vi "Auto Launch.vi"(8 "error in (no error)":errorcluster, 11 "Task in":refnum<class "Task Config.lvclass">) -> (0 "error out":errorcluster, 2 "Auto Launch":bool, 3 "Task out":refnum<class "Task Config.lvclass">)   [LabVIEW 2020, in "VolatusConfig.lvlib" / "Task Config.lvclass"]
uses:
  Task Config.lvclass
  Task Config.lvclass/Task Config.ctl
  lv-cdm/CDM-Config/Config Element/Config Element.lvclass
  VolatusConfigElement/VolatusConfigElement.lvclass
  C:/dev/lv20CE/relink/lv-volatus/VolatusConfig/VolatusConfigElement/VolatusConfigElement.lvclass
  C:/dev/lv20CE/relink/lv-volatus/VolatusConfig/Task/Task Config.lvclass
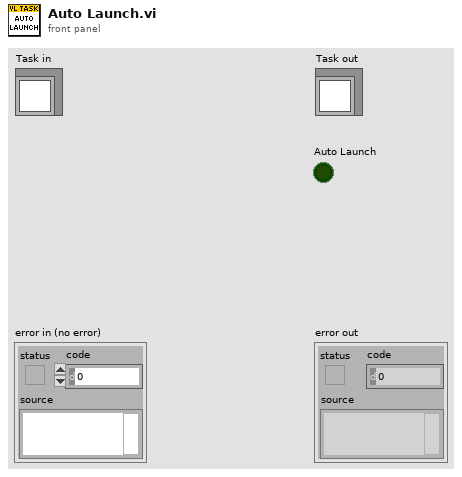
[diagram p1: front panel]
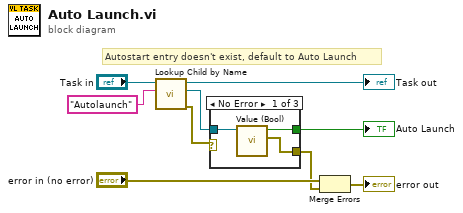
[diagram p0: block diagram]
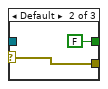
[diagram p2: hidden frame]
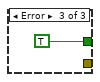
[diagram p3: hidden frame]
diagram:
  # "Autostart entry doesn't exist, default to Auto Launch"
  n1 = call "Lookup Child by Name.vi"("Child Name"="Autolaunch" ("Name"), "VolatusConfigElement in"="Task in") -> ("error out"=w2:errorcluster, "Child"=w1:refnum<class "Config Element.lvclass">, "VolatusConfigElement out"=→"Task out":refnum<class "Task Config.lvclass">)  [unwired: 6 in, 1 out]
  n2 = case shown="No Error" w2 {
    selector: w2 -> [_ w13 _]
    tunnel: [w11 FALSE ("Bool Value") TRUE] -> w7
    tunnel: w1 -> [w12 _ _]
    tunnel: [w10 w13 _] -> w5
    frame No Error {
      n3 = call "Value (Bool).vi"("Config Element in"=w12) -> ("error out"=w10:errorcluster, "Bool Value"=w11:bool)  [unwired: 9 in]
    }
    frame Default {
    }
    frame Error {
    }
  }
  "Auto Launch" <- w7
  n4 = Merge Errors("error in (no error)", w5) -> (→"error out":errorcluster)
